vi "EXCEL report.vi"(7 "Report state":T1=enum."Close report", 8 "error in":errorcluster, 10 "Data in":variant) -> (0 "error out":errorcluster, 2 "Data out":variant)   [LabVIEW 2015, in "Report.lvlib"]
uses:
  Report.lvlib
  <vilib>/Utility/NIReport.llb/NI_report.lvclass
  <vilib>/Utility/NIReport.llb/NI_ReportGenerationCore.lvlib
  <vilib>/Utility/NIReport.llb/Excel/NI_Excel.lvclass
  <vilib>/Utility/NIReport.llb/Append Text Table to Report (wrap).vi
  TypeDefs/Report state.ctl
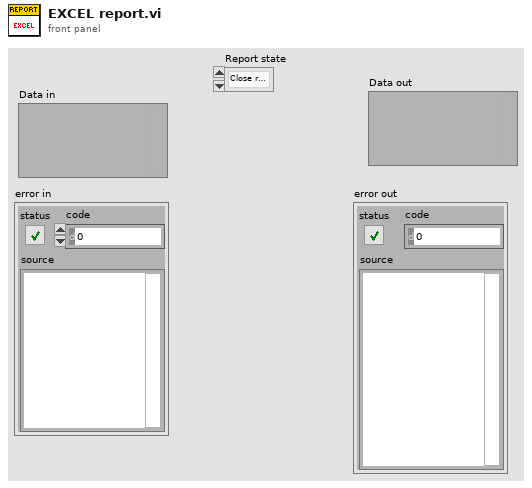
[diagram p1: front panel]
types:
  T1 = typedef "Report.lvlib/Report state.ctl" = enum16{"Create report", "Save data", "Save report", "Available printers", "Print report", "Close report"}
  T2 = enum16{"Standard Report", "HTML", "Word", "Excel"}
  T3 = enum16{"maximized", "minimized", "normal", "no change"}
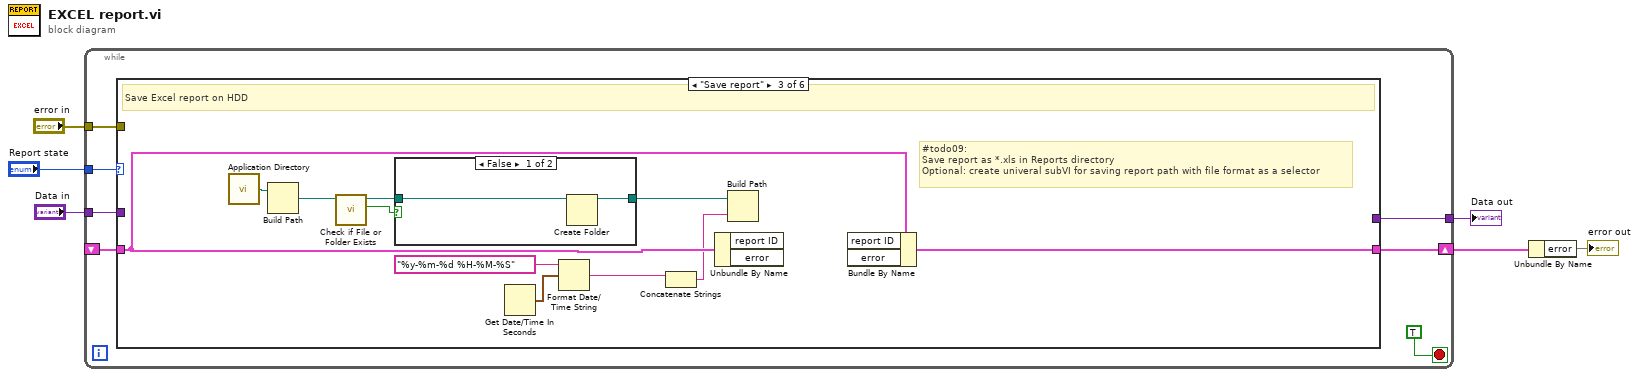
[diagram p0: block diagram]
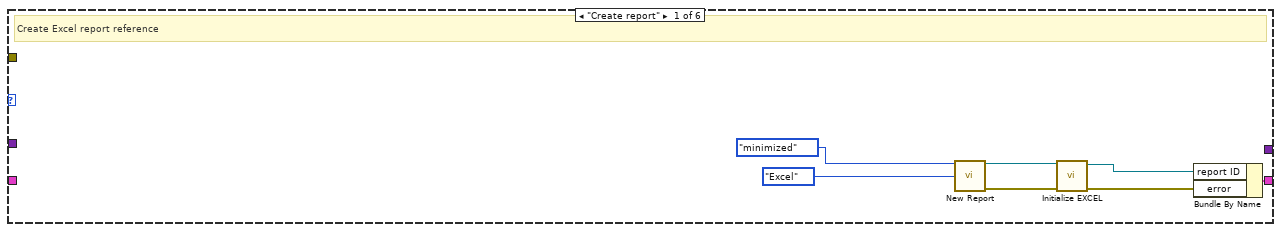
[diagram p2: hidden frame]
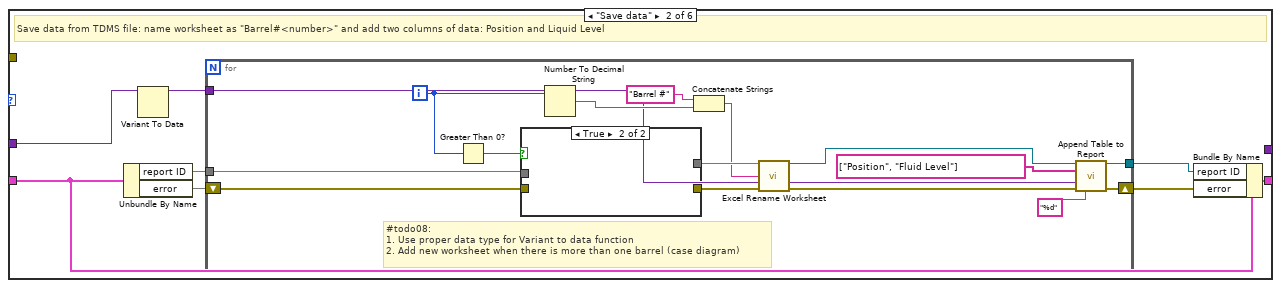
[diagram p3: hidden frame]
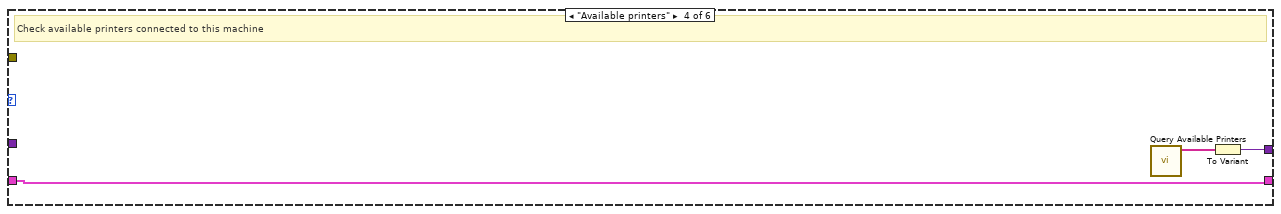
[diagram p6: hidden frame]
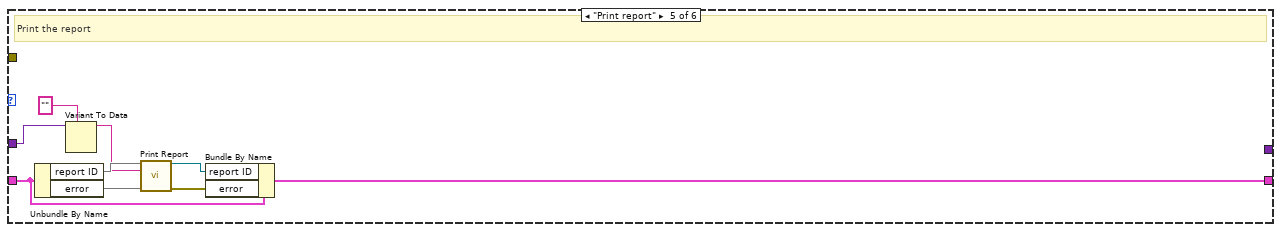
[diagram p7: hidden frame]
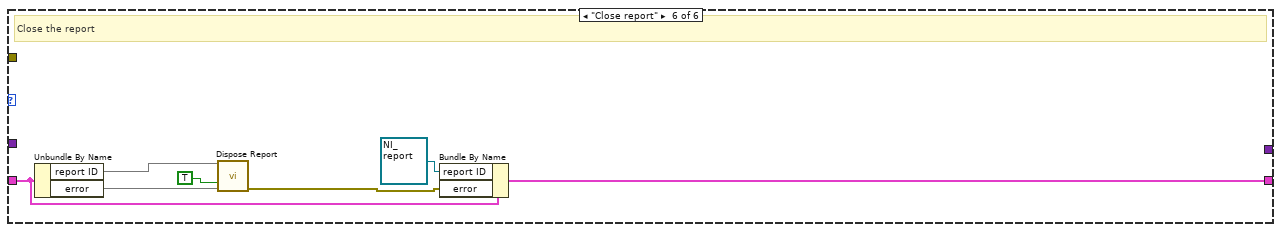
[diagram p8: hidden frame]
diagram:
  n1 = while {
    tunnel: "Report state" -> [w9]
    shift-right: [w11] -> w3
    shift-left: _ -> [w12]
    tunnel: "Data in" -> [w10]
    tunnel: "error in" -> [w8]
    tunnel: [w7] -> w1
    stop <- TRUE stop-if-true
    n2 = case shown="\"Save report\"" w9 {
      tunnel: w12 -> [_ w28 w57 w61 w70 w78]
      tunnel: [w20 w27 w56 w61 w69 w79] -> w11
      tunnel: w10 -> [_ w26 _ _ w66 _]
      tunnel: w8 -> [_ _ _ _ _ _]
      tunnel: [_ _ _ w62 _ _] -> w7
      frame "Create report" {
        # "Create Excel report reference"
        n3 = call <vilib>:"New Report.vi"("window state (normal)"=T3."minimized", "report type"=T2."Excel") -> ("report out"=w17:refnum<class "NI_report.lvclass">, "error out"=w16:errorcluster)  [unwired: 12 in]
        n4 = call "Initialize EXCEL.vi"("error in (no error)"=w16, "NI_report in"=w17) -> ("error out"=w14:errorcluster, "NI_report out"=w15:refnum<class "NI_report.lvclass">)  [unwired: 8 in]
        n5 = Bundle By Name("report ID"=w15, "error"=w14) -> (w20:cluster{})  [unwired: 1 in]
      }
      frame "Save data" {
        # "Save data from TDMS file: name worksheet as \"Barrel#<number>\" and add two columns of data: Position and Liquid Level"
        n6 = Unbundle By Name(w28) -> ("report ID"=w23, "error"=w25)
        n7 = Variant To Data(Variant=w26) -> (data=w24:variant)  [unwired: 2 in, 1 out]
        n8 = for {
          tunnel: w24 -> [w32]
          shift-right: [w33] -> w21
          shift-left: w25 -> [w39]
          tunnel: w23 -> [w40]
          tunnel: [w34] -> w22
          i -> [w41]
          # "#todo08:\n1. Use proper data type for Variant to data function\n2. Add new worksheet when there is more than one barrel (case diagram)"
          n9 = Greater Than 0?(x=w41) -> (x > 0?=w42:bool)
          n10 = case shown="True" w42 {
            tunnel: w40 -> [w46 _]
            tunnel: w39 -> [w45 _]
            tunnel: [w46 _] -> w38
            tunnel: [w45 _] -> w37
            frame False {
            }
            frame True {
            }
          }
          n11 = Number To Decimal String(number=w41) -> (decimal integer string=w43:string)  [unwired: 1 in]
          n12 = Concatenate Strings("Barrel #", w43) -> (w31:string)
          n13 = call <vilib>:"Excel Rename Worksheet.vi"("report in"=w38, "worksheet name (\"\")"=w31, "error in (no error)"=w37) -> ("report out"=w36:refnum<class "NI_report.lvclass">, "error out"=w35:errorcluster)  [unwired: 11 in]
          n14 = call-poly <vilib>:"Append Table to Report.vi"("report in"=w36, "column headers"=string[] ["Position", "Fluid Level"], "text data"=w32, "error in (no error)"=w35, 12:"%d" ("format string (%.3f)")) -> ("report out"=w34:refnum<class "NI_report.lvclass">, "error out"=w33:errorcluster)  [unwired: 7 in, 2 out]
        }
        n15 = Bundle By Name(cluster=w28, "report ID"=w22, "error"=w21) -> (w27:cluster{})
      }
      frame "Save report" {
        # "#todo09:\nSave report as *.xls in Reports directory\nOptional: create univeral subVI for saving report path with file format as a selector"
        # "Save Excel report on HDD"
        n16 = call <vilib>:"Application Directory.vi"() -> ("Application Directory"=w51:path)
        n17 = Build Path(base path=w51) -> (appended path=w50:path)  [unwired: 1 in]
        n18 = call <vilib>:"Check if File or Folder Exists.vi"("path"=w50) -> ("file or folder exists?"=w49:bool, "dup path"=w48:path)  [unwired: 8 in, 1 out]
        n19 = case shown="False" w49 {
          tunnel: w48 -> [w59 w60]
          tunnel: [w58 w60] -> w47
          frame False {
            n20 = Create Folder(path (use dialog)=w59) -> (created path=w58:path)  [unwired: 2 in, 2 out]
          }
          frame True {
          }
        }
        n21 = Get Date/Time In Seconds() -> (seconds since 1Jan1904=w55:timestamp)
        n22 = Format Date/Time String(time format string (%c)="%y-%m-%d %H-%M-%S", seconds (now)=w55) -> (date/time string=w53:string)  [unwired: 1 in]
        n23 = Concatenate Strings(w53) -> (w52:string)  [unwired: 1 in]
        n24 = Unbundle By Name(w57) -> ()  [unwired: 2 out]
        n25 = Build Path(base path=w47, name or relative path=w52) -> ()  [unwired: 1 out]
        n26 = Bundle By Name(cluster=w57) -> (w56:cluster{})  [unwired: 2 in]
      }
      frame "Available printers" {
        # "Check available printers connected to this machine"
        n27 = call <vilib>:"Query Available Printers.vi"() -> ("system configured printers"=w63:string[])  [unwired: 9 in, 2 out]
        n28 = To Variant(anything=w63) -> (Variant=w62:variant)
      }
      frame "Print report" {
        # "Print the report"
        n29 = Unbundle By Name(w70) -> ("report ID"=w72, "error"=w71)
        n30 = Variant To Data(type="", Variant=w66) -> (data=w64:string)  [unwired: 1 in, 1 out]
        n31 = call-dynamic "Print Report.vi"("report in"=w72, "printer name (default)"=w64, "error in (no error)"=w71) -> ("report out"=w68:refnum<class "NI_report.lvclass">, "error out"=w67:errorcluster)  [unwired: 11 in]
        n32 = Bundle By Name(cluster=w70, "report ID"=w68, "error"=w67) -> (w69:cluster{})
      }
      frame "Close report" {
        # "Close the report"
        n33 = Unbundle By Name(w78) -> ("report ID"=w77, "error"=w76)
        n34 = call-dynamic "Dispose Report.vi"("report in"=w77, "save changes? (F)"=TRUE, "error in (no error)"=w76) -> ("error out"=w75:errorcluster)  [unwired: 12 in]
        n35 = Bundle By Name(cluster=w78, "report ID"=refnum<class "NI_report.lvclass"> refnum ("Report ID"), "error"=w75) -> (w79:cluster{})
      }
    }
  }
  "Data out" <- w1
  n36 = Unbundle By Name(w3) -> ("error"=→"error out")
